vi "util-timer-inline.vi"(8 "Error In":errorcluster, 9 "Reset?":bool, 10 "Target[ms]":dbl) -> (0 "Error Out":errorcluster, 1 "done?":bool, 2 "ElapsedTime[sec]":dbl, 3 "downcount[sec]":dbl)   [LabVIEW 2024]
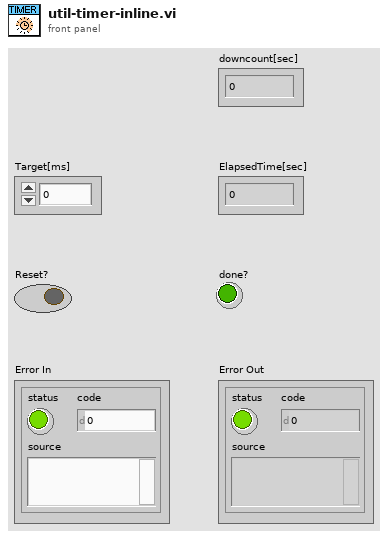
[diagram p1: front panel]
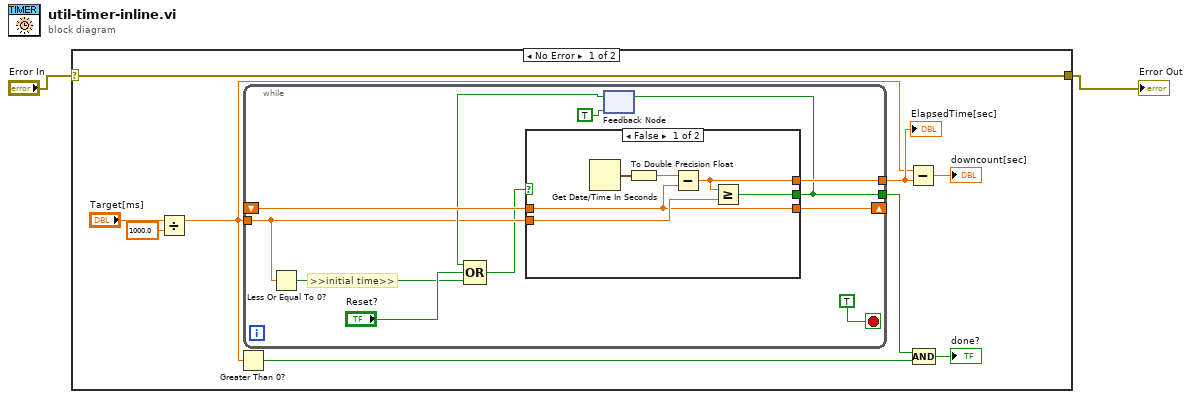
[diagram p0: block diagram]
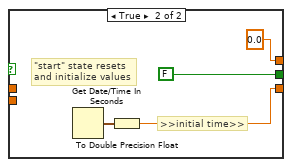
[diagram p2: hidden frame]
diagram:
  n1 = case shown="No Error" "Error In" {
    selector: "Error In" -> [w5 w33]
    tunnel: [w5 w33] -> w1
    frame No Error {
      n2 = Divide(x="Target[ms]", y=1000.0) -> (x/y=w4:dbl)
      n3 = Greater Than 0?(x=w4) -> (x > 0?=w6:bool)
      n4 = while {
        shift-right: [w21] -> _
        shift-left: _ -> [w19]
        tunnel: [w20] -> w10
        tunnel: w4 -> [w14]
        tunnel: [w18] -> w11
        stop <- TRUE stop-if-true
        # ">>initial time>>"
        n5 = Less Or Equal To 0?(x=w14) -> (x <= 0?=w13:bool)
        n6 = feedback #1(TRUE) -> (w16:bool)
        n7 = Compound Arithmetic op=OR(w16, "Reset?", w13) -> (w12:bool)
        n8 = case shown="False" w12 {
          tunnel: [w23 w29] -> w21
          tunnel: [w27 FALSE] -> w18
          tunnel: [w26 0.0 ("Elapsed Time")] -> w20
          tunnel: w19 -> [w23 _]
          tunnel: w14 -> [w28 _]
          frame False {
            n9 = Get Date/Time In Seconds() -> (seconds since 1Jan1904=w25:timestamp)
            n10 = To Double Precision Float(number=w25) -> (double precision float=w24:dbl)
            n11 = Subtract(x=w24, y=w23) -> (x-y=w26:dbl)
            n12 = Greater Or Equal?(x=w26, y=w28) -> (x >= y?=w27:bool)
          }
          frame True {
            # "\"start\" state resets \nand initialize values"
            # ">>initial time>>"
            n13 = Get Date/Time In Seconds() -> (seconds since 1Jan1904=w30:timestamp)
            n14 = To Double Precision Float(number=w30) -> (double precision float=w29:dbl)
          }
        }
        n15 = feedback-in #1(w18) -> ()
      }
      "ElapsedTime[sec]" <- w10
      n16 = Subtract(x=w4, y=w10) -> (x-y=→"downcount[sec]":dbl)
      n17 = Compound Arithmetic op=AND(w11, w6) -> (→"done?":bool)
    }
    frame Error {
    }
  }
  "Error Out" <- w1
